vi "Set Guardian_Measure SMU.vi"(5 "script name":string, 7 "Pins":string[](array[string])=["VDD"], 8 "error in (no error)":errorcluster, 10 "Published Data Ids":string[](array[string]), 11 "Semiconductor Module Context":T3) -> (0 "error Out":errorcluster)   [LabVIEW 2013]
uses:
  <vilib>/NI_TestStand_SemiconductorModule/NI_TestStand_Semiconductor_Module.lvlibp/PinMap/General/SemiconductorModuleContext.ctl
  <instrlib>/niDCPower/nidcpower.llb/niDCPower Sense.ctl
  <instrlib>/niHSDIO/niHSDIO.llb/niHSDIO_ctl Trigger Script - trigID Values (Ring).ctl
  <vilib>/NI_TestStand_SemiconductorModule/NI_TestStand_Semiconductor_Module.lvlibp
panel:
  out "R Array":dbl[][](array[numeric]) format="%#_6p"
  in  "SMU Settings":T2={"Level"=0.01, "Level Range"=0.1, "Limit"=1.0, "Limit Range"=6.0, "Sense"=1009} {"Sense" items=["Local"=1008, "Remote"=1009]}
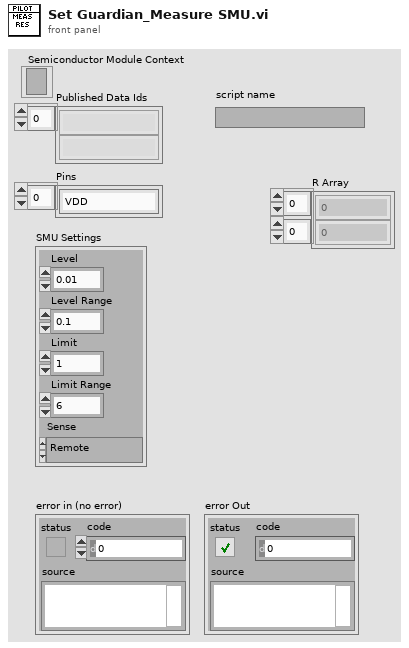
[diagram p1: front panel]
types:
  T1 = typedef "niDCPower Sense.ctl" = i32
  T2 = cluster{"Level":dbl, "Level Range":dbl, "Limit":dbl, "Limit Range":dbl, "Sense":T1}
  T3 = typedef "NI_TestStand_Semiconductor_Module.lvlibp/SemiconductorModuleContext.ctl" = refnum<k7>
  T4 = typedef "niHSDIO_ctl Trigger Script - trigID Values (Ring).ctl" = string
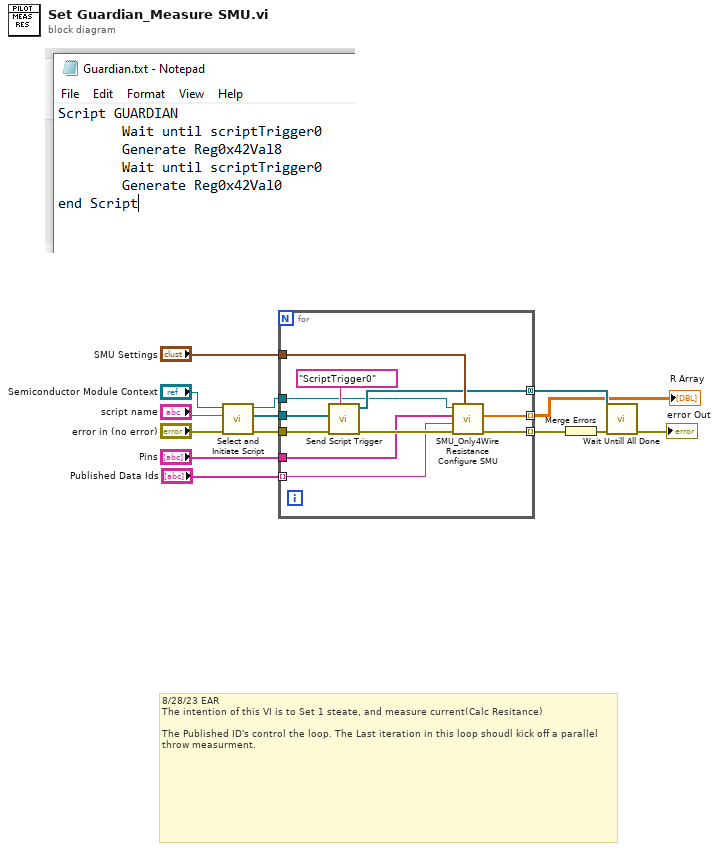
[diagram p0: block diagram]
diagram:
  # "8/28/23 EAR\nThe intention of this VI is to Set 1 steate, and measure current(Calc Resitance)\n\nThe Published ID's control the loop. The Last iteration in this loop shoudl kick off a parallel throw measurment."
  n1 = call "Select and Initiate Script.vi"("error in (no error)"="error in (no error)", "script name"="script name", "Semiconductor Module Context"="Semiconductor Module Context") -> ("error out"=w12:errorcluster, "HSDIO GEN Sessions Out"=w11:refnum<k15>[], "Semiconductor Module Context Out"=w2:T3)  [unwired: 6 in]
  n2 = for {
    tunnel: [w17] -> w6 mode=indexing
    tunnel: w12 -> [w25]
    tunnel: w11 -> [w24]
    tunnel: "SMU Settings" -> [w23]
    tunnel: "Published Data Ids" -> [w18] mode=indexing
    tunnel: "Pins" -> [w19]
    tunnel: [w16] -> w3 mode=indexing
    tunnel: [w20] -> w4 mode=concatenating
    tunnel: w2 -> [w15]
    n3 = call "Send Script Trigger.vi"("trigger id (script trigger 0)"=T4 "ScriptTrigger0", "error in (no error)"=w25, "HSDIO Sessions In"=w24) -> ("error out"=w21:errorcluster, "HSDIO Sessions Out"=w20:refnum<k15>[])  [unwired: 7 in]
    n4 = call "SMU_Only4Wire Resistance Configure SMU.vi"("SMU Settings"=w23, "error in (no error)"=w21, "Published Data Id"=w18, "Pins"=w19, "Semiconductor Module Context"=w15) -> ("error Out"=w17:errorcluster, "R Array"=w16:dbl[])  [unwired: 4 in, 1 out]
  }
  "R Array" <- w3
  n5 = Merge Errors(w6) -> (w5:errorcluster)
  n6 = call "Wait Untill All Done.vi"("error in (no error)"=w5, "HSDIO Sessions In"=w4) -> ("error out"=→"error Out":errorcluster)  [unwired: 8 in, 1 out]
